vi "Coord window-Enter offsets manually.vi"() -> (0 "error out":errorcluster)   [LabVIEW 2017]
uses:
  Globals/Coord window-Globals.vi
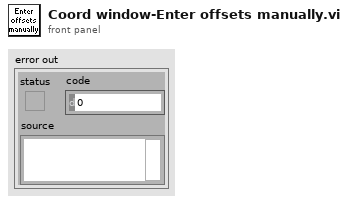
[diagram p1: front panel]
types:
  T1 = typedef "Coordinate list window refs.ctl" = cluster{"Window Name (i.e. Key)":string, "menu reference":refnum<k9>, "VI's reference":refnum<vi>, "Pane 1":refnum<vi>, "Pane 2":refnum<vi>, "Coord Listbox":refnum<vi>, "File name":refnum<vi>, "Picture Map":refnum<vi>, "Stage XYZ Position ind.":refnum<vi>}
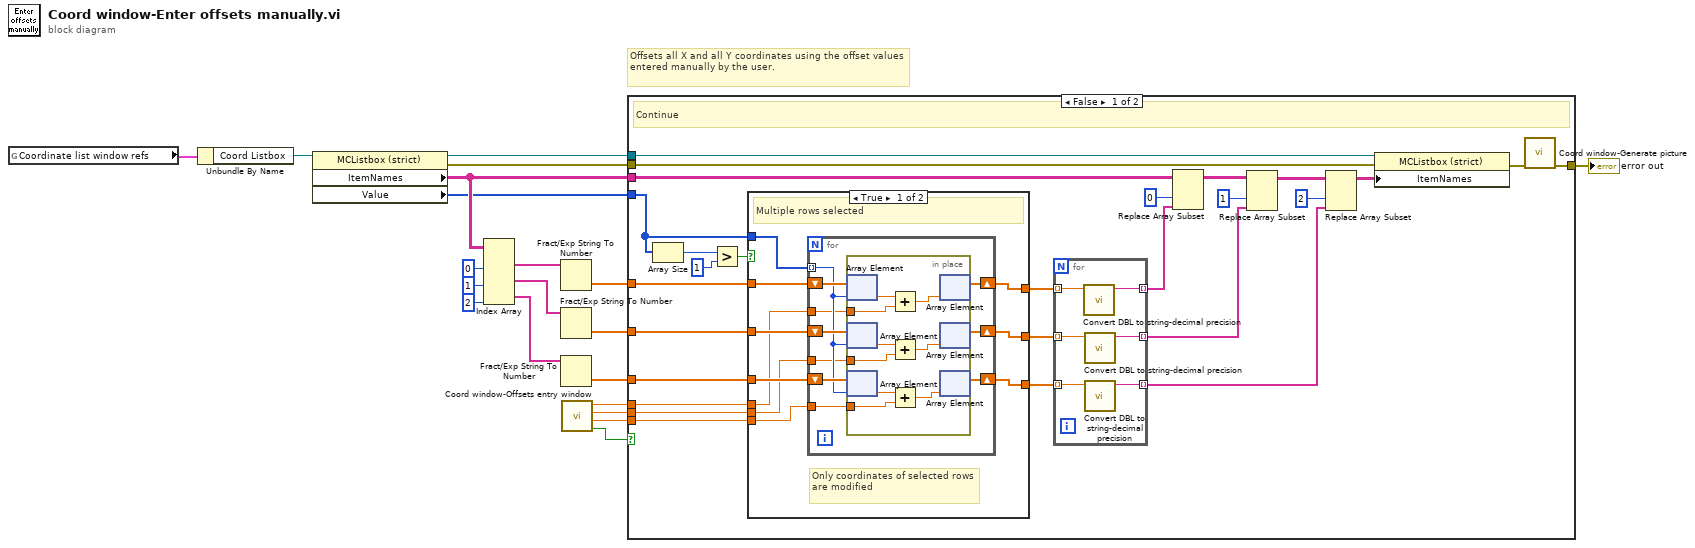
[diagram p0: block diagram]
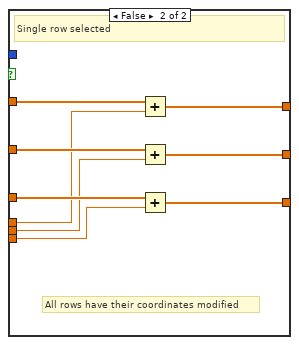
[diagram p2: hidden frame]
diagram:
  # "Offsets all X and all Y coordinates using the offset values entered manually by the user."
  n1 = global read "Coord window-Globals.vi" "Coordinate list window refs"() -> (w20:T1)
  n2 = Unbundle By Name(w20) -> ("Coord Listbox"=w19:refnum<vi>)
  n3 = property class="MCListbox (strict)"(reference=w19) -> (reference out=w11:refnum<vi>, error out=w10:errorcluster, "ItemNames"=w12:string[][], "Value"=w1:i32[])  [unwired: 1 in]
  n4 = Index Array(array=w12, index (col) #1=0 ("disabled index (col)"), index (col) #2=1 ("index (col)"), index (col) #3=2 ("index (col)")) -> (element #1=w16:string[], element #2=w15:string[], element #3=w6:string[])  [unwired: 3 in]
  n5 = Fract/Exp String To Number(string=w16) -> (number=w14:dbl[])  [unwired: 3 in, 1 out]
  n6 = Fract/Exp String To Number(string=w15) -> (number=w13:dbl[])  [unwired: 3 in, 1 out]
  n7 = Fract/Exp String To Number(string=w6) -> (number=w7:dbl[])  [unwired: 3 in, 1 out]
  n8 = call "Coord window-Offsets entry window.vi"() -> ("Cancelled"=w2:bool, "Z offset out"=w3:dbl, "Y offset out"=w4:dbl, "X offset out"=w5:dbl)  [unwired: 8 in]
  n9 = case shown="False" w2 {
    tunnel: w14 -> [w47 _]
    tunnel: w13 -> [w46 _]
    tunnel: w12 -> [w45 _]
    tunnel: w11 -> [w41 _]
    tunnel: w10 -> [w40 w92]
    tunnel: [w38 w92] -> w9
    tunnel: w7 -> [w37 _]
    tunnel: w5 -> [w33 _]
    tunnel: w4 -> [w32 _]
    tunnel: w3 -> [w31 _]
    tunnel: w1 -> [w30 _]
    frame False {
      # "Continue"
      n10 = Array Size(array=w30) -> (size(s)=w29:i32)
      n11 = Greater?(x=w29, y=1) -> (0:w28:bool)
      n12 = case shown="True" w28 {
        tunnel: w47 -> [w63 w91]
        tunnel: w46 -> [w62 w90]
        tunnel: [w55 w84] -> w25
        tunnel: [w56 w85] -> w26
        tunnel: w37 -> [w61 w89]
        tunnel: [w54 w83] -> w24
        tunnel: w33 -> [w60 w88]
        tunnel: w32 -> [w59 w87]
        tunnel: w31 -> [w58 w86]
        tunnel: w30 -> [w57 _]
        frame True {
          # "Only coordinates of selected rows are modified"
          # "Multiple rows selected"
          n13 = for {
            tunnel: w60 -> [w66]
            tunnel: w59 -> [w65]
            tunnel: w58 -> [w64]
            shift-right: [w67] -> w56
            shift-left: w63 -> [w73]
            shift-right: [w68] -> w55
            shift-left: w62 -> [w72]
            shift-right: [w69] -> w54
            shift-left: w61 -> [w71]
            tunnel: w57 -> [w70] mode=indexing
            n14 = in-place {
              in-place-border: w66 -> [w81]
              in-place-border: w65 -> [w75]
              in-place-border: w64 -> [w74]
              n15 = in-place-array #1(w73, w70) -> (w82:dbl)
              n16 = in-place-array #2(w72, w70) -> (w79:dbl)
              n17 = in-place-array #3(w71, w70) -> (w78:dbl)
              n18 = Add(x=w82, y=w81) -> (x+y=w80:dbl)
              n19 = Add(x=w79, y=w75) -> (x+y=w77:dbl)
              n20 = Add(x=w78, y=w74) -> (x+y=w76:dbl)
              n21 = in-place-array #1(w80) -> (w67:dbl[])  [unwired: 1 out]
              n22 = in-place-array #2(w77) -> (w68:dbl[])  [unwired: 1 out]
              n23 = in-place-array #3(w76) -> (w69:dbl[])  [unwired: 1 out]
            }
          }
        }
        frame False {
          # "All rows have their coordinates modified"
          # "Single row selected"
          n24 = Add(x=w91, y=w88) -> (x+y=w85:dbl[])
          n25 = Add(x=w90, y=w87) -> (x+y=w84:dbl[])
          n26 = Add(x=w89, y=w86) -> (x+y=w83:dbl[])
        }
      }
      n27 = for {
        tunnel: w26 -> [w53] mode=indexing
        tunnel: w25 -> [w52] mode=indexing
        tunnel: [w51] -> w23 mode=indexing
        tunnel: [w50] -> w22 mode=indexing
        tunnel: w24 -> [w48] mode=indexing
        tunnel: [w49] -> w21 mode=indexing
        n28 = call <userlib>:"Convert DBL to string-decimal precision.vi"("DBL Value"=w53) -> ("Converted to String"=w51:string)  [unwired: 10 in]
        n29 = call <userlib>:"Convert DBL to string-decimal precision.vi"("DBL Value"=w52) -> ("Converted to String"=w50:string)  [unwired: 10 in]
        n30 = call <userlib>:"Convert DBL to string-decimal precision.vi"("DBL Value"=w48) -> ("Converted to String"=w49:string)  [unwired: 10 in]
      }
      n31 = Replace Array Subset(array=w45, new element=w23, index (col)=0 ("disabled index (col)")) -> (w43:string[][])  [unwired: 1 in]
      n32 = Replace Array Subset(array=w43, new element=w22, index (col)=1 ("disabled index (col)")) -> (w35:string[][])  [unwired: 1 in]
      n33 = Replace Array Subset(array=w35, new element=w21, index (col)=2 ("disabled index (col)")) -> (w34:string[][])  [unwired: 1 in]
      n34 = property class="MCListbox (strict)"(reference=w41, error in=w40, "ItemNames"=w34) -> (error out=w39:errorcluster)  [unwired: 1 out]
      n35 = call "Coord window-Generate picture.vi"("error in (no error)"=w39) -> ("error out"=w38:errorcluster)  [unwired: 10 in]
    }
    frame True {
      # "Cancelled"
    }
  }
  "error out" <- w9
